vi "Init SPI.vi"(8 "error in (no error)":errorcluster, 10 "DMA FIFO ref in":refnum<k20>, 11 "Device Ref in":T1 format="%.0x") -> (0 "error out":errorcluster, 1 "Compiled Info":T2 {"Current Sense Engine Data"."Ordered Channels" format="%.0x"; "Current Sense Engine Data"."RT IDs"."Slot #" max=15; "Current Sense Engine Data"."RT IDs"."Chip Address (A2 A1 A0)" max=7; "Resistor Engine Data"."Ordered Channels" format="%.0x"; "Resistor Engine Data"."RT IDs"."Slot #" max=15; "Resistor Engine Data"."RT IDs"."Chip Address (A2 A1 A0)" max=7; "Wheel Speed Sensor Engine Data"."Ordered Channels" format="%.0x"; "Wheel Speed Sensor Engine Data"."RT IDs"."Slot #" max=15; "Wheel Speed Sensor Engine Data"."RT IDs"."Chip Address (A2 A1 A0)" max=7; "Battery Switch Engine Data"."Ordered Channels" format="%.0x"; "Battery Switch Engine Data"."RT IDs"."Slot #" max=15; "Battery Switch Engine Data"."RT IDs"."Chip Address (A2 A1 A0)" max=7; "FIU Engine Data"."Ordered Channels" format="%.0x"; "FIU Engine Data"."RT IDs"."Slot #" max=15; "FIU Engine Data"."RT IDs"."Chip Address (A2 A1 A0)" max=7}, 2 "DMA FIFO ref out":refnum<k20>, 3 "Device Ref out":T1 format="%.0x")   [LabVIEW 2014, in "SLSC configuration Engine.lvlib"]
uses:
  SLSC configuration Engine.lvlib
  <vilib>/NI Veristand/Custom Device API/Custom Device Item Ref.ctl
  Shared/Type Defs/SLSC compiled.ctl
  Shared/Type Defs/Res Sim compiled.ctl
  Shared/Type Defs/RT Engine Data.ctl
  Shared/Type Defs/RT IDs.ctl
  Shared/SPI Utility/Slot #.ctl
  Shared/MCP23S17/Chip Address.ctl
  Shared/Constants.vi
  <vilib>/NI Veristand/Custom Device API/Get Item Property (Variant).vi
  <vilib>/Utility/error.llb/Error Cluster From Error Code.vi
  <vilib>/rvi/errors/niLvFpgaAdjustHostInterfaceError.vi
  <vilib>/rvi/interface/nirviMethod/nirviMethod.xnode
  <vilib>/NI Veristand/Custom Device API/Custom Device API.lvlib
  Shared/SLSC configuration Shared.lvlib
  <vilib>/FPGAPlugInAG/Dynamic/niLvFpga_WriteFifo_Dynamic.vi
  <vilib>/rvi/errors/niLvFpgaMergeErrorWithErrorCode.vi
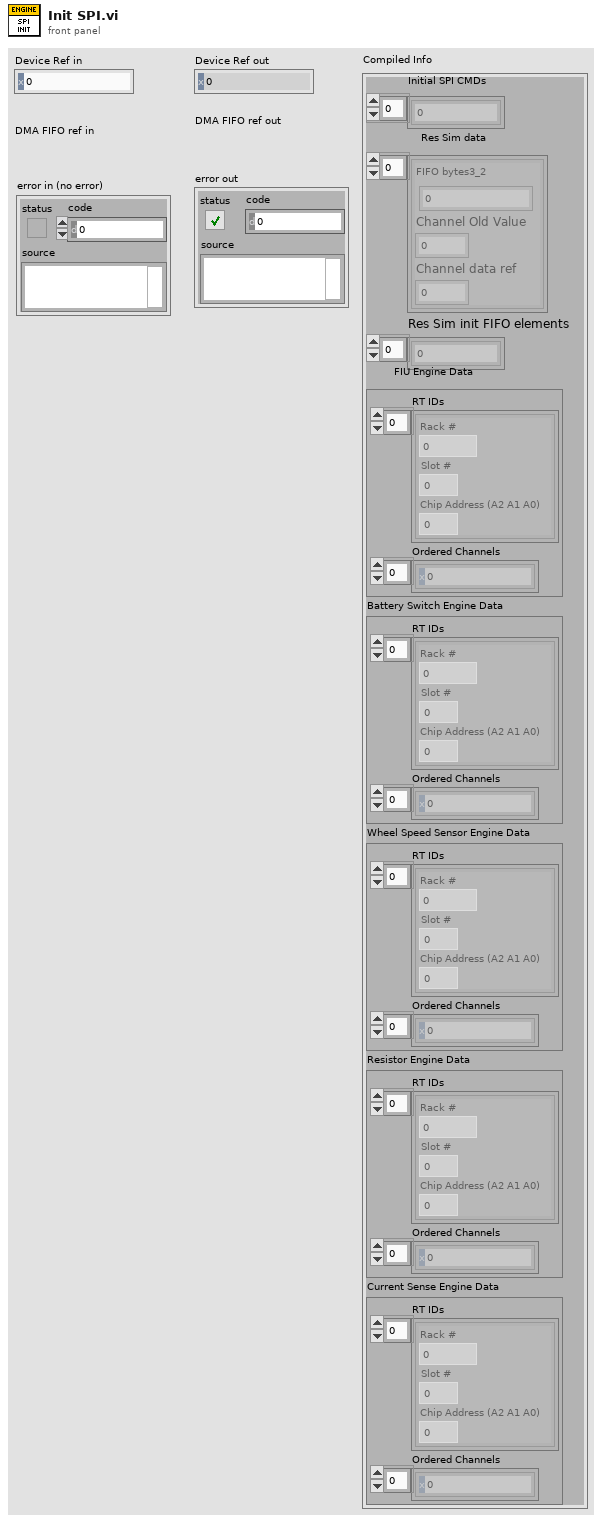
[diagram p1: front panel]
types:
  T1 = typedef "Custom Device API.lvlib/Custom Device Item Ref.ctl" = u64
  T2 = typedef "SLSC configuration Shared.lvlib/SLSC compiled.ctl" = cluster{"Initial SPI CMDs":u64[], "Res Sim data ":T3[], "Res Sim init FIFO elements":u32[], "FIU Engine Data":T4, "Battery Switch Engine Data":T4, "Wheel Speed Sensor Engine Data":T4, "Resistor Engine Data":T4, "Current Sense Engine Data":T4}
  T3 = typedef "SLSC configuration Shared.lvlib/Res Sim compiled.ctl" = cluster{"FIFO bytes3_2":u16, "Channel Old Value":dbl, "Channel data ref":i32}
  T4 = typedef "SLSC configuration Shared.lvlib/RT Engine Data.ctl" = cluster{"RT IDs":T5[], "Ordered Channels":T1[]}
  T5 = typedef "SLSC configuration Shared.lvlib/RT IDs.ctl" = cluster{"Rack #":u8, "Slot #":T6, "Chip Address (A2 A1 A0)":T7}
  T6 = typedef "SLSC configuration Shared.lvlib/Slot #.ctl" = u8
  T7 = typedef "SLSC configuration Shared.lvlib/Chip Address.ctl" = u8
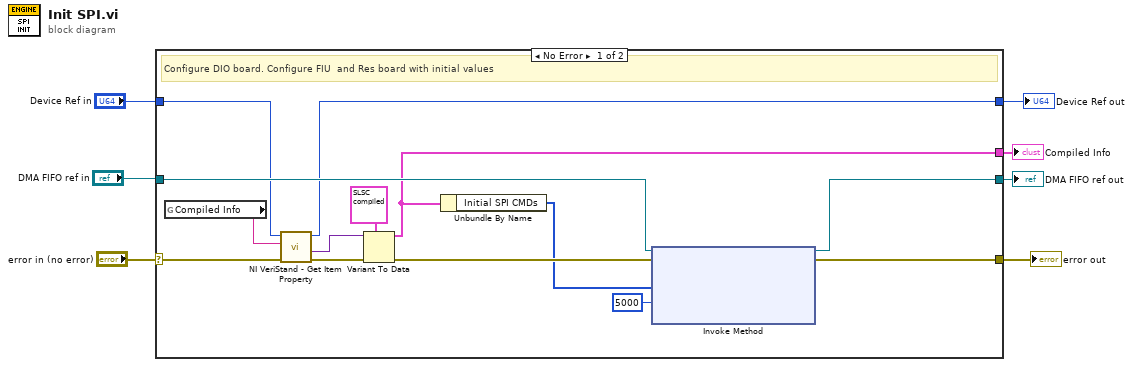
[diagram p0: block diagram]
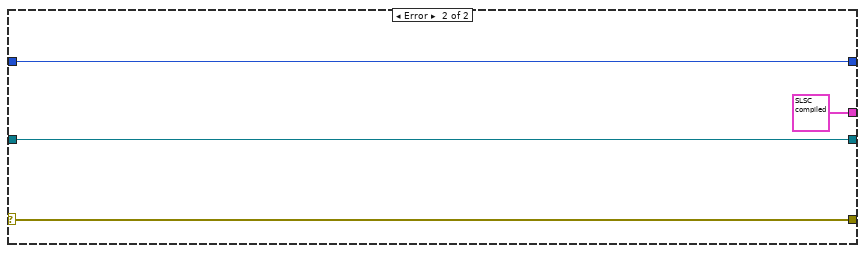
[diagram p2: hidden frame]
diagram:
  n1 = case shown="No Error" "error in (no error)" {
    selector: "error in (no error)" -> [w12 w24]
    tunnel: "DMA FIFO ref in" -> [w16 w25]
    tunnel: [w14 w25] -> w2
    tunnel: [w10 w24] -> w7
    tunnel: "Device Ref in" -> [w13 w22]
    tunnel: [w11 T2 {"Initial SPI CMDs"=[], "Res Sim data "=[], "Res Sim init FIFO elements"=[], "FIU Engine Data"={"RT IDs"=[], "Ordered Channels"=[]}, "Battery Switch Engine Data"={"RT IDs"=[], "Ordered Channels"=[]}, "Wheel Speed Sensor Engine Data"={"RT IDs"=[], "Ordered Channels"=[]}, "Resistor Engine Data"={"RT IDs"=[], "Ordered Channels"=[]}, "Current Sense Engine Data"={"RT IDs"=[], "Ordered Channels"=[]}} ("type")] -> w4
    tunnel: [w8 w22] -> w1
    frame No Error {
      # "Configure DIO board. Configure FIU  and Res board with initial values"
      n2 = global read "Constants.vi" "Compiled Info"() -> (w21:string)
      n3 = call-poly <vilib>:"NI VeriStand - Get Item Property.vi"("error in (no error)"=w12, "Property Name"=w21, "Item Ref in"=w13) -> ("error out"=w20:errorcluster, "Value"=w19:variant, "Item Ref out"=w8:T1)  [unwired: 5 in, 1 out]
      n4 = Variant To Data(error in=w20, type=T2 {"Initial SPI CMDs"=[], "Res Sim data "=[], "Res Sim init FIFO elements"=[], "FIU Engine Data"={"RT IDs"=[], "Ordered Channels"=[]}, "Battery Switch Engine Data"={"RT IDs"=[], "Ordered Channels"=[]}, "Wheel Speed Sensor Engine Data"={"RT IDs"=[], "Ordered Channels"=[]}, "Resistor Engine Data"={"RT IDs"=[], "Ordered Channels"=[]}, "Current Sense Engine Data"={"RT IDs"=[], "Ordered Channels"=[]}}, Variant=w19) -> (data=w11:T2, error out=w17:errorcluster)
      n5 = Unbundle By Name(w11) -> ("Initial SPI CMDs"=w9:u64[])
      n6 = xnode "Invoke Method"("FPGA VI Reference In"=w16, "error in"=w17, "Data"=w9, "Timeout (ms)"=5000) -> ("FPGA VI Reference Out"=w14:refnum<k20>, "error out"=w10:errorcluster)  [unwired: 1 out]
    }
    frame Error {
    }
  }
  "error out" <- w7
  "Compiled Info" <- w4
  "DMA FIFO ref out" <- w2
  "Device Ref out" <- w1
